vi "lm Shut Down.vi"(8 "error in (no error)":errorcluster, 11 "hSerial":u32) -> (0 "error out":errorcluster, 3 "hSerial out":u32)   [LabVIEW 2015, in "LumencorDLL32.lvlib"]
doc: "This function closes the current com port and releases it for other applications.\n\nextern \"C\" LUMENCORDLL2B_API void lmShutDown(HANDLE hSerial);"
uses:
  <userlib>/LumencorDLL32/LumencorDLL32.lvlib
  <userlib>/LumencorDLL32/LumencorDLL32.dll
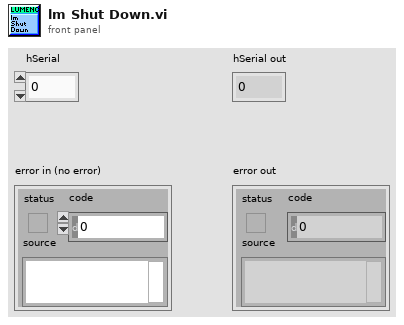
[diagram p1: front panel]
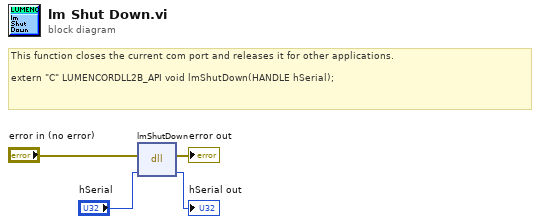
[diagram p0: block diagram]
diagram:
  # "This function closes the current com port and releases it for other applications.\n\nextern \"C\" LUMENCORDLL2B_API void lmShutDown(HANDLE hSerial);"
  n1 = dll-call lib="C:/Program Files (x86)/National Instruments/LabVIEW 2015/user.lib/LumencorDLL32/LumencorDLL32.*" fn="lmShutDown"(error in="error in (no error)", "hSerial"="hSerial") -> (error out=→"error out":errorcluster, "hSerial"=→"hSerial out":u32)  [unwired: 3 in, 1 out]
